vi "APC_RunHRL_inPC.vi"() -> ()   [LabVIEW 2020]
uses:
  controls/APC_CombustionMetrics.ctl
  controls/APC_PcylDiag.ctl
  <vilib>/Utility/file.llb/Read Delimited Spreadsheet (DBL).vi
panel:
  out "PcylDiagWarningsAndErrors":T1[](array[typedef])
  out "Q":dbl[][](graph)
  out "HP filtered":dbl[][](graph)
  in  "Manual":bool
  in  "Manual cycle":i32
  in  "Expected IMEP":dbl
  in  "millisecond multiple":u32
  out "cycle":i32
  out "PreIgnition":bool
  out "element":string="C:\\Carlos\\OneDrive - UPV\\B-Propuestas\\NOBLE\\2023 MONARCH\\1.-INFO\\PressureTraces\\knock\\20230404_145426_C9SingleCyl_TEST130_CA60Cycles.txt"
  in  "test":i32=10
  in  "stop":bool
  out "Pressures":dbl[][](graph)
  out "CombustionAnalysisCluster":T2={"IMEPn [bar]"=[6.211117999242393, 6.211117999242393, 6.211117999242393, 6.211117999242393, 6.211117999242393, 6.211117999242393], "IMEPg [bar]"=[6.4446479514403014, 6.4446479514403014, 6.4446479514403014, 6.4446479514403014, 6.4446479514403014, 6.4446479514403014], "MAPO [bar/CAD]"=[12.032314460918599, 12.032314460918599, 12.032314460918599, 12.032314460918599, 12.032314460918599, 12.032314460918599], "maxQ [J]"=[1738.4237704292323, 1738.4237704292323, 1738.4237704292323, 1738.4237704292323, 1738.4237704292323, 1738.4237704292323], "CA10  [CADATDC]"=[-3.3498503358307232, -3.3498503358307232, -3.3498503358307232, -3.3498503358307232, -3.3498503358307232, -3.3498503358307232], "CA50 [CADATDC]"=[5.494620967564458, 5.494620967564458, 5.494620967564458, 5.494620967564458, 5.494620967564458, 5.494620967564458], "CA90 [CADATDC]"=[nan, nan, nan, nan, nan, nan], "Pmax [bar]"=[65.51369273351828, 65.51369273351828, 65.51369273351828, 65.51369273351828, 65.51369273351828, 65.51369273351828], "IMEPstd [bar]"=[0.1430846822513861, 0.1430846822513861, 0.1430846822513861, 0.1430846822513861, 0.1430846822513861, 0.1430846822513861], "CA03  [CADATDC]"=[nan, nan, nan, nan, nan, nan], "CA97  [CADATDC]"=[nan, nan, nan, nan, nan, nan], "CA10CA90 [CADATDC]"=[nan, nan, nan, nan, nan, nan], "maxdpdCAD [bar/CAD]"=[nan, nan, nan, nan, nan, nan], "kappa_comp [-]"=[nan, nan, nan, nan, nan, nan], "kappa_exp [-]"=[nan, nan, nan, nan, nan, nan], "PMEP [bar]"=[nan, nan, nan, nan, nan, nan], "RI [-]"=[nan, nan, nan, nan, nan, nan]}
  out "prechamber pressure":dbl[](array[numeric])
  out "6 P cyl example":dbl[][](array[numeric])
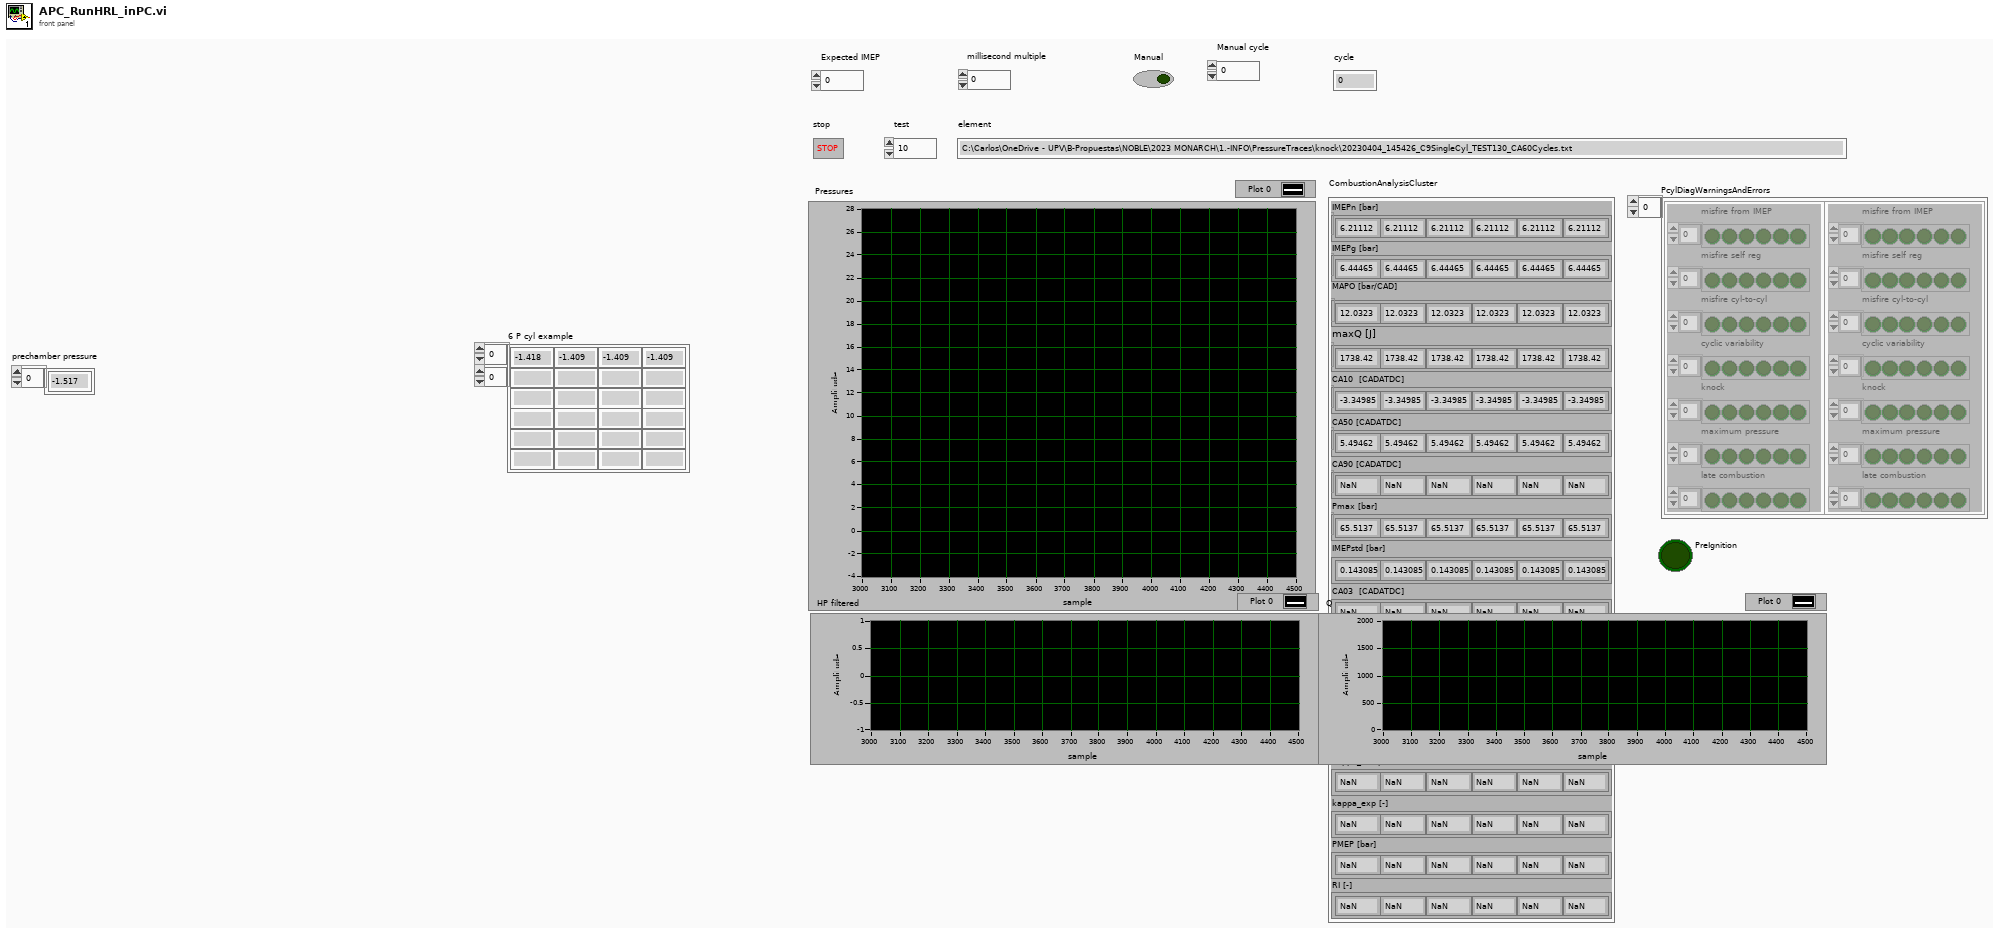
[diagram p1: front panel]
types:
  T1 = typedef "APC_PcylDiag.ctl" = cluster{"misfire from IMEP":bool[], "misfire self reg":bool[], "misfire cyl-to-cyl":bool[], "cyclic variability":bool[], "knock":bool[], "maximum pressure":bool[], "late combustion":bool[]}
  T2 = typedef "APC_CombustionMetrics.ctl" = cluster{"IMEPn [bar]":dbl[], "IMEPg [bar]":dbl[], "MAPO [bar/CAD]":dbl[], "maxQ [J]":dbl[], "CA10  [CADATDC]":dbl[], "CA50 [CADATDC]":dbl[], "CA90 [CADATDC]":dbl[], "Pmax [bar]":dbl[], "IMEPstd [bar]":dbl[], "CA03  [CADATDC]":dbl[], "CA97  [CADATDC]":dbl[], "CA10CA90 [CADATDC]":dbl[], "maxdpdCAD [bar/CAD]":dbl[], "kappa_comp [-]":dbl[], "kappa_exp [-]":dbl[], "PMEP [bar]":dbl[], "RI [-]":dbl[]}
  T3 = cluster{"IIR LowPass":cluster{"filter structure":enum32{"IIR 2nd Order", "IIR 4th Order"}, "Reverse Coefficients":dbl[], "Forward Coefficients":dbl[]}, "IIR HighPass":cluster{"filter structure":enum32{"IIR 2nd Order", "IIR 4th Order"}, "Reverse Coefficients":dbl[], "Forward Coefficients":dbl[]}}
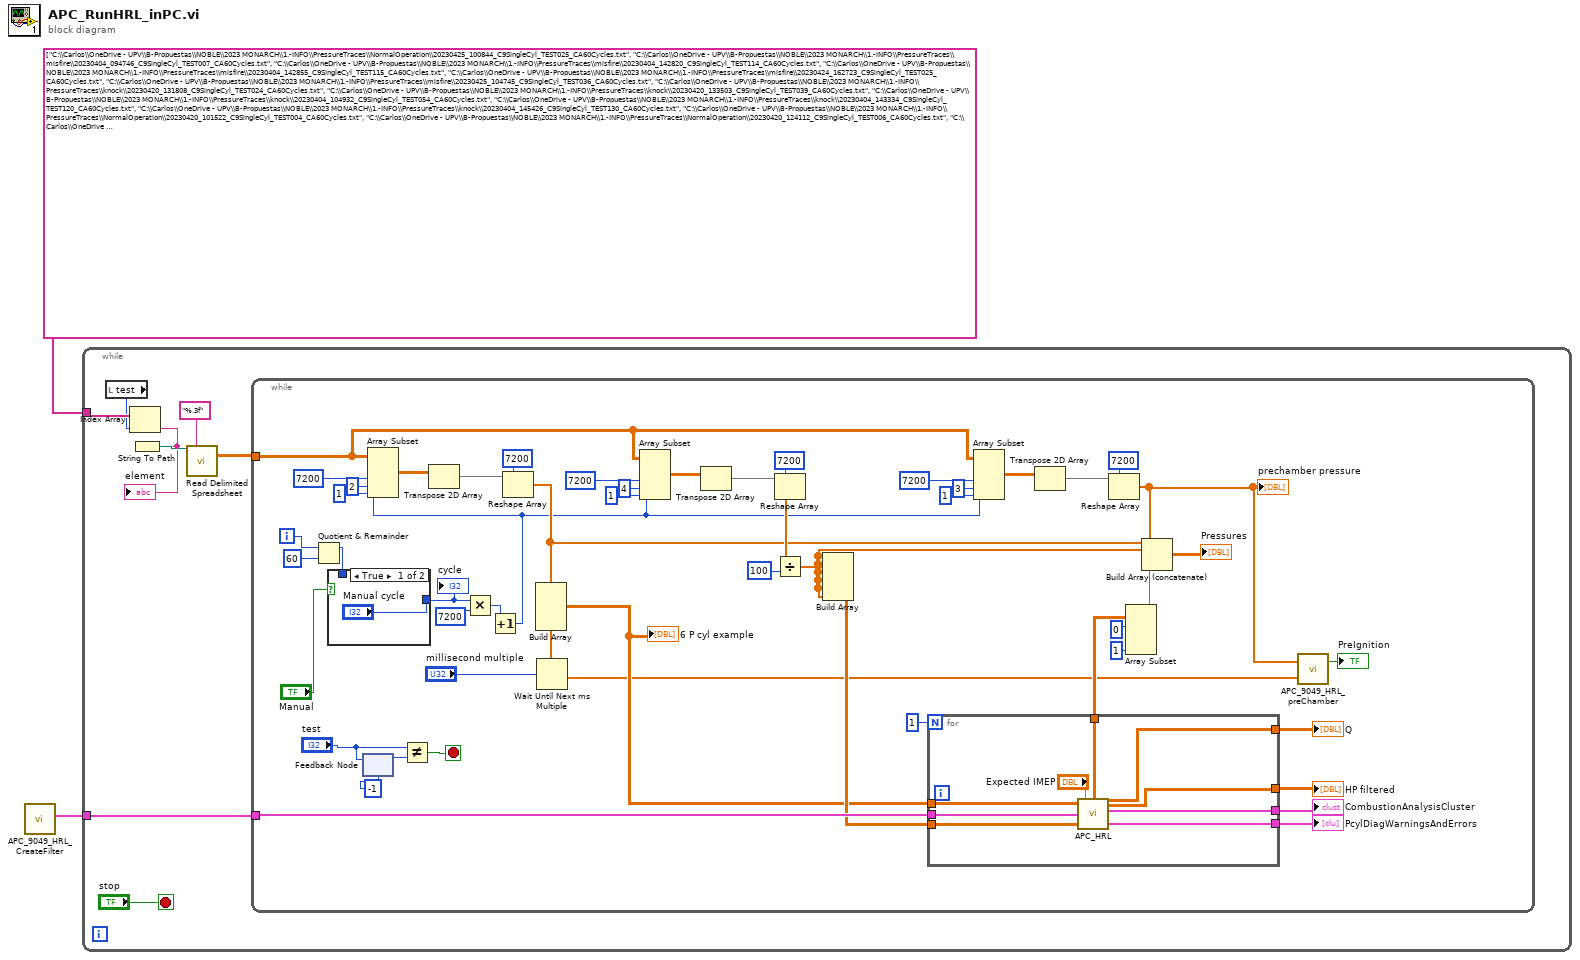
[diagram p0: block diagram]
diagram:
  n1 = call "APC_9049_HRL_CreateFilter.vi"() -> ("FilterCoefs"=w2:T3)  [unwired: 11 in]
  n2 = while {
    tunnel: w2 -> [w10]
    tunnel: string[] ["C:\\Carlos\\OneDrive - UPV\\B-Propuestas\\NOBLE\\2023 MONARCH\\1.-INFO\\PressureTraces\\NormalOperation\\20230425_100844_C9SingleCyl_TEST025_CA60Cycles.txt", "C:\\Carlos\\OneDrive - UPV\\B-Propuestas\\NOBLE\\2023 MONARCH\\1.-INFO\\PressureTraces\\misfire\\20230404_094746_C9SingleCyl_TEST007_CA60Cycles.txt", "C:\\Carlos\\OneDrive - UPV\\B-Propuestas\\NOBLE\\2023 MONARCH\\1.-INFO\\PressureTraces\\misfire\\20230404_142820_C9SingleCyl_TEST114_CA60Cycles.txt", "C:\\Carlos\\OneDrive - UPV\\B-Propuestas\\NOBLE\\2023 MONARCH\\1.-INFO\\PressureTraces\\misfire\\20230404_142855_C9SingleCyl_TEST115_CA60Cycles.txt", "C:\\Carlos\\OneDrive - UPV\\B-Propuestas\\NOBLE\\2023 MONARCH\\1.-INFO\\PressureTraces\\misfire\\20230424_162723_C9SingleCyl_TEST025_CA60Cycles.txt", "C:\\Carlos\\OneDrive - UPV\\B-Propuestas\\NOBLE\\2023 MONARCH\\1.-INFO\\PressureTraces\\misfire\\20230425_104745_C9SingleCyl_TEST036_CA60Cycles.txt", "C:\\Carlos\\OneDrive - UPV\\B-Propuestas\\NOBLE\\2023 MONARCH\\1.-INFO\\PressureTraces\\knock\\20230420_131808_C9SingleCyl_TEST024_CA60Cycles.txt", "C:\\Carlos\\OneDrive - UPV\\B-Propuestas\\NOBLE\\2023 MONARCH\\1.-INFO\\PressureTraces\\knock\\20230420_133503_C9SingleCyl_TEST039_CA60Cycles.txt", "C:\\Carlos\\OneDrive - UPV\\B-Propuestas\\NOBLE\\2023 MONARCH\\1.-INFO\\PressureTraces\\knock\\20230404_104932_C9SingleCyl_TEST054_CA60Cycles.txt", "C:\\Carlos\\OneDrive - UPV\\B-Propuestas\\NOBLE\\2023 MONARCH\\1.-INFO\\PressureTraces\\knock\\20230404_143334_C9SingleCyl_TEST120_CA60Cycles.txt", "C:\\Carlos\\OneDrive - UPV\\B-Propuestas\\NOBLE\\2023 MONARCH\\1.-INFO\\PressureTraces\\knock\\20230404_145426_C9SingleCyl_TEST130_CA60Cycles.txt", "C:\\Carlos\\OneDrive - UPV\\B-Propuestas\\NOBLE\\2023 MONARCH\\1.-INFO\\PressureTraces\\NormalOperation\\20230420_101522_C9SingleCyl_TEST004_CA60Cycles.txt", "C:\\Carlos\\OneDrive - UPV\\B-Propuestas\\NOBLE\\2023 MONARCH\\1.-INFO\\PressureTraces\\NormalOperation\\20230420_124112_C9SingleCyl_TEST006_CA60Cycles.txt", "C:\\Carlos\\OneDrive - UPV\\B-Propuestas\\NOBLE\\2023 MONARCH\\1.-INFO\\PressureTraces\\NormalOperation\\20230502_123958_C9SingleCyl_TEST076_CA60Cycles.txt", "C:\\Carlos\\OneDrive - UPV\\B-Propuestas\\NOBLE\\2023 MONARCH\\1.-INFO\\PressureTraces\\NormalOperation\\20230502_124531_C9SingleCyl_TEST077_CA60Cycles.txt"] -> [w8]
    stop <- "stop" stop-if-true
    n3 = local read "test"() -> (w5:i32)
    n4 = Index Array(array=w8, index=w5) -> (element=w6:string)
    "element" <- w6
    n5 = String To Path(string=w6) -> (path=w7:path)
    n6 = call-poly <vilib>:"Read Delimited Spreadsheet.vi"("file path (dialog if empty)"=w7, "format (%.3f)"="%.3f") -> ("all rows"=w4:dbl[][])  [unwired: 8 in, 5 out]
    n7 = while {
      tunnel: w10 -> [w61]
      tunnel: w4 -> [w24]
      i -> [w23]
      stop <- w25 stop-if-true
      n8 = Quotient & Remainder(x=w23, y=60) -> (x-y*floor(x/y)=w16:i32)  [unwired: 1 out]
      n9 = case shown="True" "Manual" {
        tunnel: w16 -> [_ w63]
        tunnel: ["Manual cycle" w63] -> w15
        frame True {
        }
        frame False {
        }
      }
      "cycle" <- w15
      n10 = feedback #1(-1 ("test")) -> (w31:i32)
      n11 = feedback-in #1("test") -> ()
      n12 = Not Equal?(x="test", y=w31) -> (x != y?=w25:bool)
      n13 = Multiply(x=w15, y=7200 ("length")) -> (x*y=w32:i32)
      n14 = Increment(x=w32) -> (x+1=w19:i32)
      n15 = Array Subset(array=w24, index (row)=w19, length (row)=7200 ("length"), index (col)=2 ("index"), length (col)=1 ("length")) -> (w57:dbl[][])
      n16 = Transpose 2D Array(2D array=w57) -> (transposed array=w56:dbl[][])
      n17 = Reshape Array(w56, 7200 ("dimension size")) -> (w20:dbl[])
      n18 = Build Array(w20, w20, w20, w20, w20, w20) -> (w27:dbl[][])
      "6 P cyl example" <- w27
      n19 = Wait Until Next ms Multiple(millisecond multiple="millisecond multiple") -> ()  [unwired: 1 out]
      n20 = Array Subset(array=w24, index (row)=w19, length (row)=7200 ("length"), index (col)=4 ("index"), length (col)=1 ("length")) -> (w51:dbl[][])
      n21 = Transpose 2D Array(2D array=w51) -> (transposed array=w50:dbl[][])
      n22 = Reshape Array(w50, 7200 ("dimension size")) -> (w28:dbl[])
      n23 = Divide(x=w28, y=100 ("length")) -> (x/y=w37:dbl[])
      n24 = Build Array(w37, w37, w37, w37, w37, w37) -> (w41:dbl[][])
      n25 = for {
        N: 1 -> [_]
        tunnel: w61 -> [w72]
        tunnel: w27 -> [w68]
        tunnel: w41 -> [w67]
        tunnel: [w71] -> w39
        tunnel: [w70] -> w36
        tunnel: [w69] -> w11
        tunnel: [w65] -> w13
        tunnel: [w64] -> w12
        n26 = call "APC_HRL.vi"("Pcyl"=w68, "exhaust pressure"=w67, "FilterCoefs"=w72, "Expected IMEP"="Expected IMEP") -> ("LPfilt Pcyl"=w70:dbl[][], "HRL [J]"=w64:dbl[][], "CombustionAnalysisCluster"=w71:T2, "HPfilt Pcyl"=w65:dbl[][], "PcylDiagWarningsAndErrors"=w69:T1[])
      }
      "CombustionAnalysisCluster" <- w39
      "HP filtered" <- w13
      "Q" <- w12
      "PcylDiagWarningsAndErrors" <- w11
      n27 = Array Subset(array=w24, index (row)=w19, length (row)=7200 ("length"), index (col)=3 ("index"), length (col)=1 ("length")) -> (w44:dbl[][])
      n28 = Transpose 2D Array(2D array=w44) -> (transposed array=w43:dbl[][])
      n29 = Reshape Array(w43, 7200 ("dimension size")) -> (w21:dbl[])
      "prechamber pressure" <- w21
      n30 = Array Subset(array=w36, index (row)=0 ("index"), length (row)=1 ("length")) -> (w26:dbl[][])  [unwired: 2 in]
      n31 = Build Array (concatenate)(w20, w37, w26, w21) -> (→"Pressures":dbl[][])
      n32 = call "APC_9049_HRL_preChamber.vi"("InCylPressure"=w20, "PrechamberPressure"=w21) -> ("PreIgnition"=→"PreIgnition":bool)  [unwired: 1 out]
    }
  }
